vi "Path to Example Theme--constant.vi"() -> (3 "Path to Example Theme":path)   [LabVIEW 2021, in "Material SubVIs.lvlib"]
doc: "CONSTANT VI - defines a default path to one of the installed themes\n\nUsed when first installing tool and opening up material editor so that it populates something from the start!\n\n<b>Code Developed By:</b> +\nDaniel Coons +\nTechnology Service Corporation +\nwww.tsc.com/atcs"
uses:
  Material SubVIs.lvlib
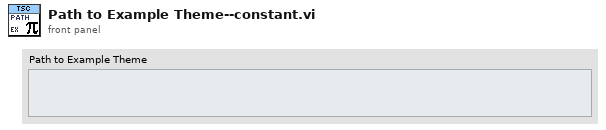
[diagram p1: front panel]
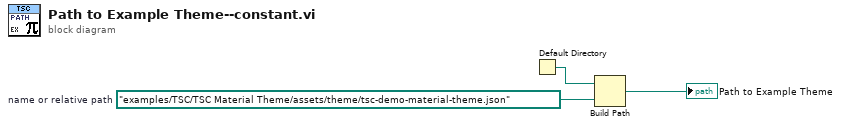
[diagram p0: block diagram]
diagram:
  w3 = path "examples/TSC/TSC Material Theme/assets/theme/tsc-demo-material-theme.json"  # name or relative path
  n1 = Default Directory() -> (w1:path)
  n2 = Build Path(base path=w1, name or relative path=w3) -> (appended path=→"Path to Example Theme":path)
